vi "Data_processing.vi"(4 "Presssure":T2, 5 "Auxiliary":T3 {"EOS" items=["Ideal", "CH4_van_der_Waal", "CH4_Redlich_Kwong", "CO2_van_der_Waal", "CO2_Redlich_Kwong", ""]}) -> (0 "z":dbl, 1 "Latest Data":T1 {"Pressure (barg)" scale=0.0..70.0}, 2 "V_v (ml)":dbl, 3 "rho_bulk":dbl)   [LabVIEW 2016]
uses:
  auxiliary_cluster.ctl
  EOS.ctl
  pressure_cluster.ctl
  adsorbed_cluster.ctl
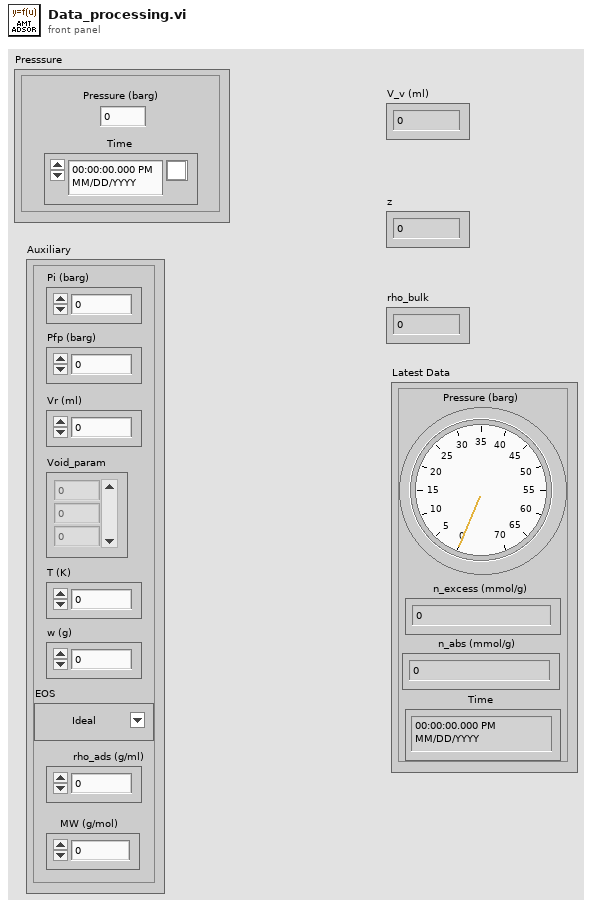
[diagram p1: front panel]
types:
  T1 = typedef "adsorbed_cluster.ctl" = cluster{"Time":timestamp, "Pressure (barg)":dbl, "n_excess (mmol/g)":dbl, "n_abs (mmol/g)":dbl}
  T2 = typedef "pressure_cluster.ctl" = cluster{"Time":timestamp, "Pressure (barg)":dbl}
  T3 = typedef "auxiliary_cluster.ctl" = cluster{"Pi (barg)":dbl, "Pfp (barg)":dbl, "Vr (ml)":dbl, "T (K)":dbl, "w (g)":dbl, "Void_param":dbl[], "EOS":T4, "rho_ads (g/ml)":dbl, "MW (g/mol)":dbl}
  T4 = typedef "EOS.ctl" = u16
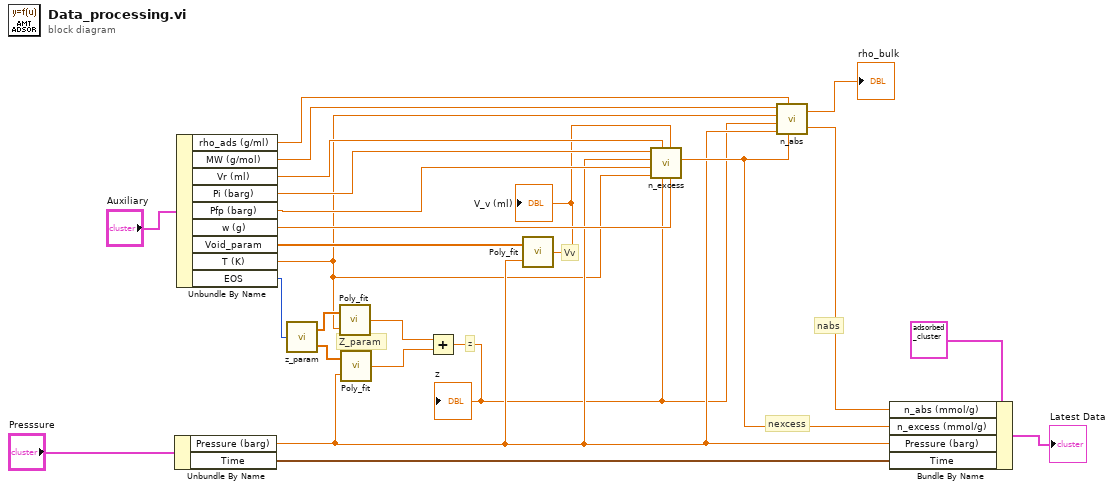
[diagram p0: block diagram]
diagram:
  # "nabs"
  # "nexcess"
  # "Z_param"
  # "z"
  # "Vv"
  n1 = Unbundle By Name("Presssure") -> ("Pressure (barg)"=w7:dbl, "Time"=w22:timestamp)
  n2 = Unbundle By Name("Auxiliary") -> ("rho_ads (g/ml)"=w3:dbl, "MW (g/mol)"=w4:dbl, "Vr (ml)"=w10:dbl, "Pi (barg)"=w11:dbl, "Pfp (barg)"=w12:dbl, "w (g)"=w13:dbl, "Void_param"=w14:dbl[], "T (K)"=w5:dbl, "EOS"=w17:T4)
  n3 = call "z_param.vi"("EOS"=w17) -> ("z_Param_T"=w19:dbl[], "z_Param_P"=w18:dbl[])
  n4 = call "Poly_fit.vi"("Input"=w5, "Parameters"=w19) -> ("Output"=w15:dbl)
  n5 = call "Poly_fit.vi"("Input"=w7, "Parameters"=w18) -> ("Output"=w16:dbl)
  n6 = Add(x=w15, y=w16) -> (x+y=w6:dbl)
  "z" <- w6
  n7 = call "Poly_fit.vi"("Input"=w7, "Parameters"=w14) -> ("Output"=w9:dbl)
  "V_v (ml)" <- w9
  n8 = call "n_excess.vi"("w"=w13, "Vv"=w9, "z"=w6, "Vr"=w10, "T"=w5, "Pfp"=w12, "Pf"=w7, "Pi"=w11) -> ("nexcess"=w8:dbl)  [unwired: 3 in]
  n9 = call "n_abs.vi"("n_excess"=w8, "rho_ads"=w3, "Pf"=w7, "z"=w6, "T"=w5, "MW"=w4) -> ("n_abs"=w1:dbl, "rho_bulk"=→"rho_bulk":dbl)
  n10 = Bundle By Name(cluster=T1 {"Time"=timestamp(0 s since 1904-01-01), "Pressure (barg)"=0.0, "n_excess (mmol/g)"=0.0, "n_abs (mmol/g)"=0.0} ("Adsorbed"), "n_abs (mmol/g)"=w1, "n_excess (mmol/g)"=w8, "Pressure (barg)"=w7, "Time"=w22) -> (→"Latest Data":T1)
